vi "UIOpen.vi"   [LabVIEW 2014, in "UILib.lvlib"]
uses:
  UILib.lvlib
  UIRefs.ctl
  <vilib>/Rock Robotics/WPI/Joystick/WPI_JoystickDeviceEnum.ctl
types:
  T1 = typedef "WPI_JoystickDeviceEnum.ctl" = enum16{"USB 0", "USB 1", "USB 2", "USB 3", "USB 4", "USB 5"}
  T2 = typedef "UILib.lvlib/UIRefs.ctl" = enum16{"Joystick0Ref", "Joystick1Ref", "Joystick2Ref"}
  T3 = typedef "WPI_JoystickDevRef.ctl" = cluster{"Device":T1}
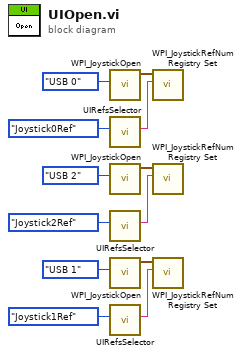
[diagram p0: block diagram]
diagram:
  n1 = call <vilib>:"WPI_JoystickOpen.vi"("JoystickDevice"=WPI_JoystickDeviceEnum."USB 0") -> ("JoystickDevRef"=w11:T3)  [unwired: 10 in]
  n2 = call "UIRefsSelector.vi"("Enum 2"=UIRefs."Joystick0Ref" ("Enum")) -> ("String"=w9:string)  [unwired: 10 in]
  n3 = call <vilib>:"WPI_JoystickOpen.vi"("JoystickDevice"=WPI_JoystickDeviceEnum."USB 2") -> ("JoystickDevRef"=w3:T3)  [unwired: 10 in]
  n4 = call "UIRefsSelector.vi"("Enum 2"=UIRefs."Joystick2Ref" ("Enum")) -> ("String"=w1:string)  [unwired: 10 in]
  n5 = call <vilib>:"WPI_JoystickOpen.vi"("JoystickDevice"=WPI_JoystickDeviceEnum."USB 1") -> ("JoystickDevRef"=w6:T3)  [unwired: 10 in]
  n6 = call "UIRefsSelector.vi"("Enum 2"=UIRefs."Joystick1Ref" ("Enum")) -> ("String"=w8:string)  [unwired: 10 in]
  n7 = call <vilib>:"WPI_JoystickRefNum Registry Set.vi"("refnum name"=w9, "JoystickDevRef"=w11) -> ()  [unwired: 8 in, 2 out]
  n8 = call <vilib>:"WPI_JoystickRefNum Registry Set.vi"("refnum name"=w1, "JoystickDevRef"=w3) -> ()  [unwired: 8 in, 2 out]
  n9 = call <vilib>:"WPI_JoystickRefNum Registry Set.vi"("refnum name"=w8, "JoystickDevRef"=w6) -> ()  [unwired: 8 in, 2 out]
